vi "KLD.vi"(0 "System no.":i32=1 min=1 max=4 step=1, 1 "Name":string, 2 "Axes to set":string[](array[string]), 3 "Position values":dbl[](array[numeric]) format="%.6f", 4 "No.of digits":i16=4, 5 "error in":errorcluster) -> (19 "error out":errorcluster)   [LabVIEW 2020]
doc: "Defines a levelling coordinate system (KLD-type) and queries ERR?. A coordinate system defined with this command is intended to eliminate hexapod misalignment. Use KLD in case misalignment is known via an external measurable deviation.\nIf there is already a coordinate system with the same name, KLD will replace it if it is not used. Activating a KLD type coordinate system (\"KEN.vi\") does not cause any motion, and \"POS?.vi\" will report new position values. If the hexapod is moving, the command cannot be applied. All pivot point coordinates (SPI.vi) will remain unchanged. SPI.vi is allowed when a KLD type coordinate system is active. For new or replaced KLD type coordinate systems, the parent coordinate system will be set to \"PI_LEVELLING\". When replacing an existing coordinate system of this type, the chain relations will be changed and the parent will be set to \"PI_LEVELLING\". For axes which are not given the position values will be set to 0. Coordinate system settings are volatile but can be saved as power-on default with WPA.vi using the password \"SKS\". This command requires command level 1 (CCL.vi). \n\nC-887, F-206, M-8X0: Only for GCS syntax version = GCS 2.0 or higher (Check with CSV?.vi. If CSV?.vi is not supported, syntax version is GCS 1.0)."
panel:
  # "Defines a levelling coordinate system (KLD-type) and queries ERR?. A \ncoordinate system defined with this command is intended to eliminate \nHexapod misalignment. Use KLD in case misalignment is known via an \nexternal measurable deviation."
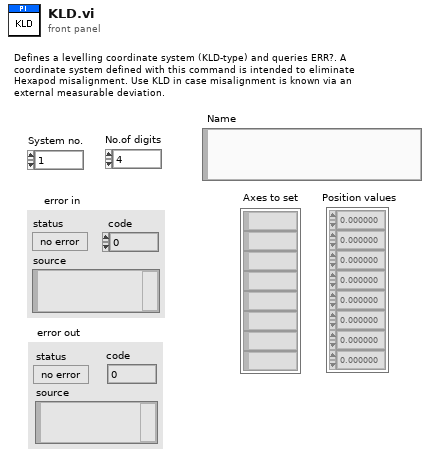
[diagram p1: front panel]
types:
  T1 = enum16{"Disable error check", "Force error check", "Use global settings"}
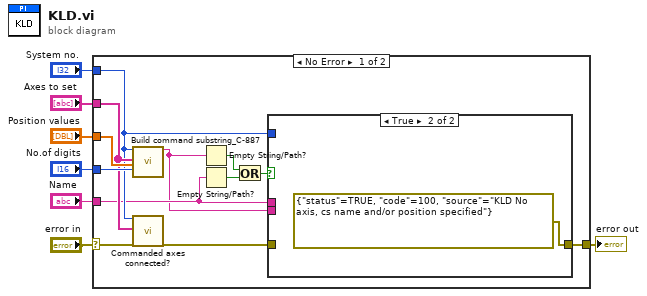
[diagram p0: block diagram]
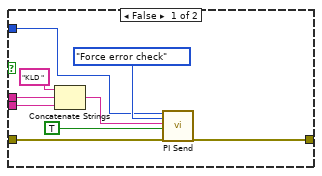
[diagram p2: hidden frame]
diagram:
  n1 = case shown="No Error" "error in" {
    selector: "error in" -> [w9 w30]
    tunnel: [w19 w30] -> w7
    tunnel: "Position values" -> [w18 _]
    tunnel: "No.of digits" -> [w17 _]
    tunnel: "System no." -> [w14 _]
    tunnel: "Axes to set" -> [w15 _]
    tunnel: "Name" -> [w13 _]
    frame No Error {
      n2 = call "Build command substring_C-887.vi"("System no."=w14, "Affected axes"=w15, "Parameters"=w18, "No. of digits"=w17) -> ("Command substring"=w8:string)  [unwired: 3 in, 12 out]
      n3 = call "Commanded axes connected?.vi"("System no."=w14, "Commanded axes"=w15, "error in"=w9) -> ("error out"=w16:errorcluster)  [unwired: 1 in, 15 out]
      n4 = Empty String/Path?(string/path=w8) -> (empty?=w12:bool)
      n5 = Empty String/Path?(string/path=w13) -> (empty?=w11:bool)
      n6 = Or(x=w12, y=w11) -> (x .or. y?=w10:bool)
      n7 = case shown="True" w10 {
        tunnel: [w22 errorcluster {"status"=TRUE, "code"=100, "source"="KLD No axis, cs name and/or position specified"} ("error out")] -> w19
        tunnel: w8 -> [w28 _]
        tunnel: w16 -> [w27 _]
        tunnel: w14 -> [w20 _]
        tunnel: w13 -> [w23 _]
        frame False {
          n8 = Concatenate Strings("KLD ", w23, w28) -> (w25:string)
          n9 = call "PI Send.vi"("System no."=w20, "Error check settings"=T1."Force error check", "String to send"=w25, "Attach termination char.?"=TRUE ("Attach Linefeed?"), "error in"=w27) -> ("error out"=w22:errorcluster)  [unwired: 1 in, 13 out]
        }
        frame True {
        }
      }
    }
    frame Error {
    }
  }
  "error out" <- w7
